vi "TSLIN Open.vi"(0 "路径输入":path, 5 "LINcount":i32(ring)=1 items=["1通道"=1, "2通道"=2, "3通道"=3, "4通道"=4, "5通道"=5], 9 "SetNodeFuntiontype":i32[](array[ring]) items=["MasterNode", "SlaveNode", "MonitorNote"], 11 "错误输入（无错误）":errorcluster) -> (4 "路径输出":path, 8 "Connect_TSLIN_Successfully":bool, 15 "错误输出":errorcluster)   [LabVIEW 2013]
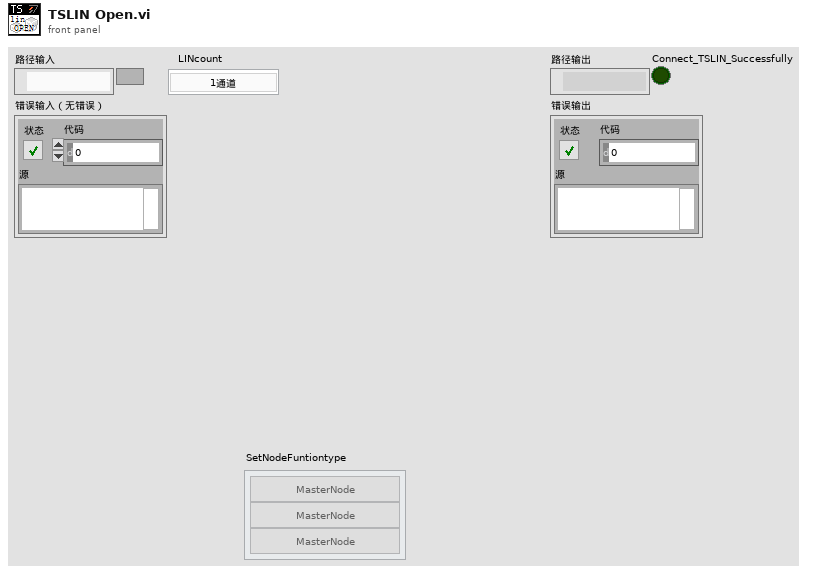
[diagram p1: front panel]
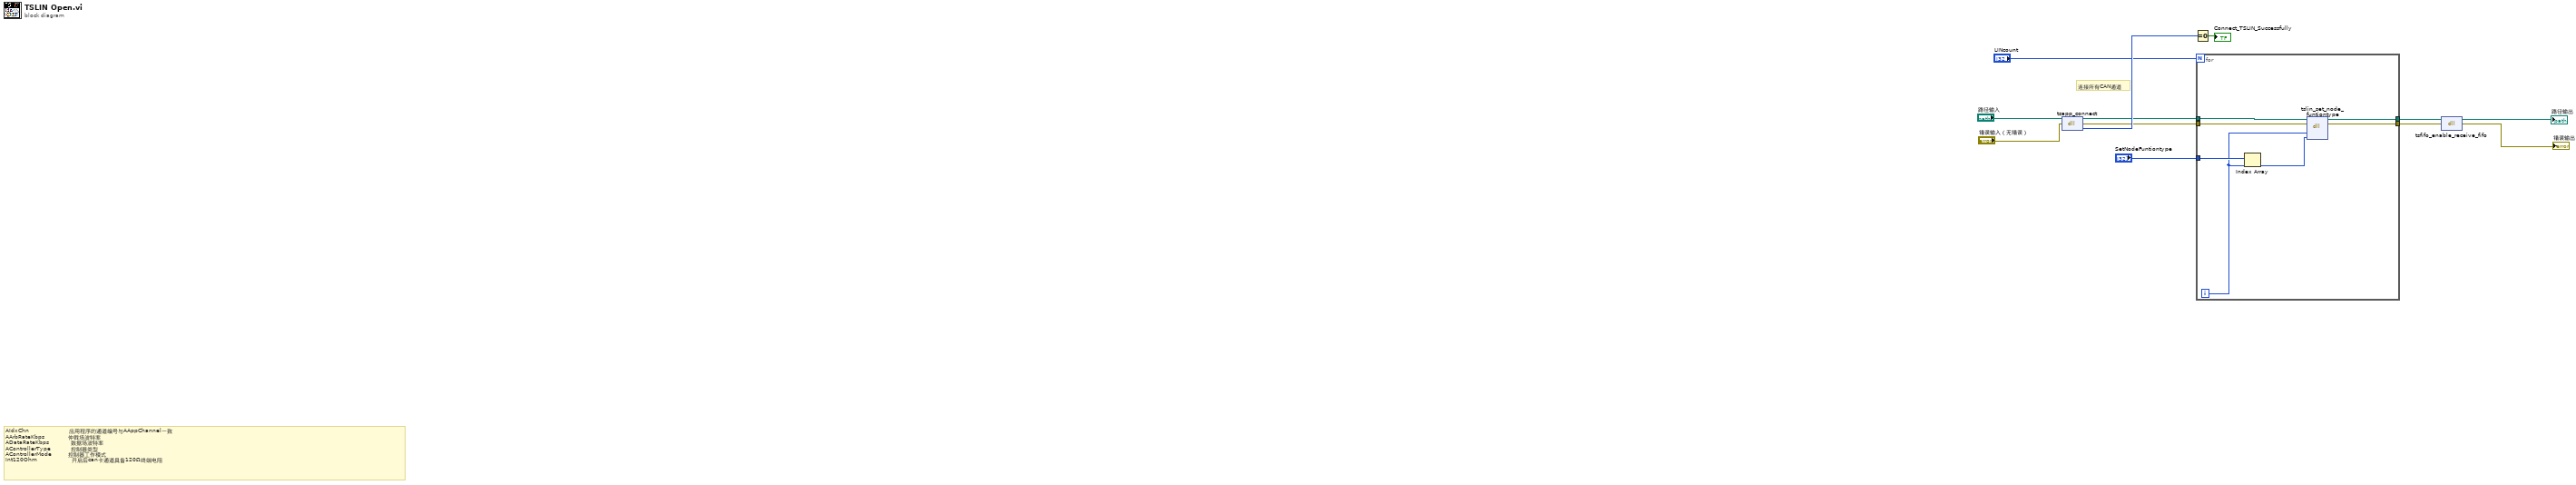
[diagram p0: block diagram]
diagram:
  # "AIdxChn                      应用程序的通道编号与AAppChannel一致\nAArbRateKbps             仲裁场波特率\nADataRateKbps            数据场波特率\nAControllerType           控制器类型\nAControllerMode         控制器工作模式\nInt120Ohm                   开启后can卡通道具备120Ω终端电阻"
  # "连接所有CAN通道"
  n1 = dll-call lib="PTH1Habs CUsers\nAdministratorDesktopTS_Can通讯PathTSMaster.dll" fn="tsapp_connect"(path in="路径输入", error in="错误输入（无错误）") -> (path out=w6:path, error out=w1:errorcluster, "tsapp_connect"=w11:i32)  [unwired: 1 in]
  n2 = Equal To 0?(x=w11) -> (x = 0?=→"Connect_TSLIN_Successfully":bool)
  n3 = for {
    N: "LINcount" -> [_]
    tunnel: w6 -> [w19]
    tunnel: [w18] -> w5
    tunnel: "SetNodeFuntiontype" -> [w17]
    tunnel: [w14] -> w2
    tunnel: w1 -> [w13]
    i -> [w16]
    n4 = Index Array(array=w17, index=w16) -> (element=w15:i32)
    n5 = dll-call lib="PTH1@abs EDemo同星TSCAN_V1.4_20220301ConfigTSMaster.dll" fn="tslin_set_node_funtiontype"(path in=w19, error in=w13, "AChnIdx"=w16, "AFunctionType"=w15) -> (path out=w18:path, error out=w14:errorcluster)  [unwired: 4 in]
  }
  n6 = dll-call lib="PTH1Habs CUsers\nAdministratorDesktopTS_Can通讯PathTSMaster.dll" fn="tsfifo_enable_receive_fifo"(path in=w5, error in=w2) -> (path out=→"路径输出":path, error out=→"错误输出":errorcluster)  [unwired: 2 in]
